vi "h.ACQ.ParseGetSpectrumData.vi"(2 "Data from #GetSpectrum":u8[](array[numeric]), 3 "power scales and offsets":i32[][](array[numeric])) -> (0 "Spectral Data":T1 {"Spectrum"."Spectrum, db" format="%_8g"})   [LabVIEW 2019, in "h.Library.lvlib"]
doc: "This vi parses the data from the h.DAQ.GetSpectrum.vi and returns a SpectralData cluster that contains the transfered peaks data.\n\n<b>Data from #GetSpectrm</b> - The data returned by the #GetSpectrum command\n<b>Spectral Data</b> - cluster containing the spectral data and supporting information"
uses:
  h.Library.lvlib
  CTL/h.ACQ.SpectralData.ctl
  CTL/h.ACQ.Spectrum.ctl
panel:
  # "Hyperion Parse Spectral Data"
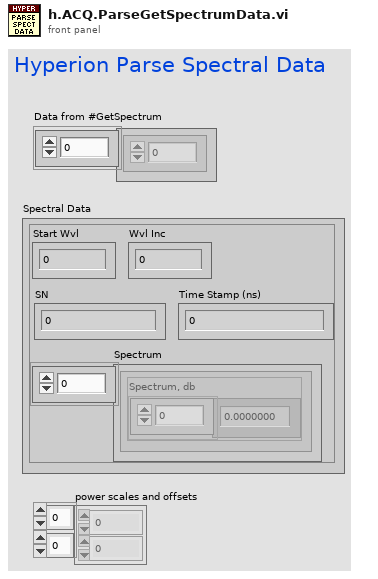
[diagram p1: front panel]
types:
  T1 = typedef "h.Library.lvlib/h.ACQ.SpectralData.ctl" = cluster{"Spectrum":T2[], "Start Wvl":dbl, "Wvl Inc":dbl, "SN":u64, "Time Stamp (ns)":u64}
  T2 = typedef "h.Library.lvlib/h.ACQ.Spectrum.ctl" = cluster{"Spectrum, db":dbl[]}
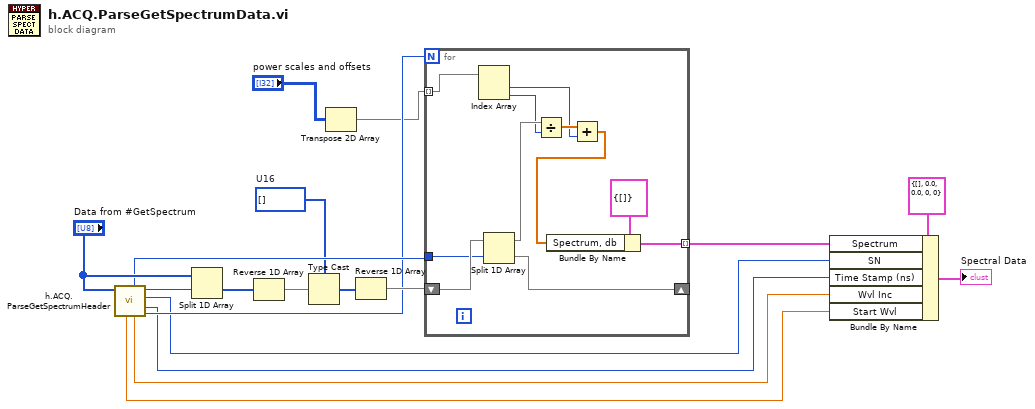
[diagram p0: block diagram]
diagram:
  w3 = u16[] []  # U16
  n1 = call "h.ACQ.ParseGetSpectrumHeader.vi"("Header from #GetSpectrum"="Data from #GetSpectrum") -> ("Channels"=w10:u16, "Time Stamp (ns)"=w7:u64, "SN"=w8:u64, "Header Length"=w15:u16, "Wvl Inc"=w6:dbl, "Num Points"=w14:u32, "Start Wvl"=w5:dbl)  [unwired: 4 in]
  n2 = Split 1D Array(array="Data from #GetSpectrum", index=w15) -> (second subarray=w4:u8[])  [unwired: 1 out]
  n3 = Reverse 1D Array(array=w4) -> (reversed array=w12:u8[])
  n4 = Type Cast(type=w3, x=w12) -> (*(type *) &x=w13:u16[])
  n5 = Transpose 2D Array(2D array="power scales and offsets") -> (transposed array=w1:i32[][])
  n6 = Reverse 1D Array(array=w13) -> (reversed array=w11:u16[])
  n7 = for {
    N: w10 -> [_]
    tunnel: w14 -> [w28]
    shift-right: [w27] -> _
    shift-left: w11 -> [w29]
    tunnel: [w25] -> w9 mode=indexing
    tunnel: w1 -> [w21] mode=indexing
    n8 = Index Array(array=w21) -> (element #1=w20:i32, element #2=w19:i32)  [unwired: 2 in]
    n9 = Split 1D Array(array=w29, index=w28) -> (first subarray=w24:u16[], second subarray=w27:u16[])
    n10 = Divide(x=w24, y=w19) -> (x/y=w22:dbl[])
    n11 = Add(x=w22, y=w20) -> (x+y=w23:dbl[])
    n12 = Bundle By Name(cluster=T2 {"Spectrum, db"=[]} ("Spectrum"), "Spectrum, db"=w23) -> (w25:T2)
  }
  n13 = Bundle By Name(cluster=T1 {"Spectrum"=[], "Start Wvl"=0.0, "Wvl Inc"=0.0, "SN"=0, "Time Stamp (ns)"=0} ("Paresed Spectral Data"), "Spectrum"=w9, "SN"=w8, "Time Stamp (ns)"=w7, "Wvl Inc"=w6, "Start Wvl"=w5) -> (→"Spectral Data":T1)
